vi "ToBoolean.vi"(8 "error in":errorcluster, 11 "Generic in":refnum<class "Generic.lvclass">) -> (0 "error out":errorcluster, 3 "Boolean out":refnum<class "Boolean.lvclass">)   [LabVIEW 2014, in "Boolean.lvclass"]
uses:
  Boolean.lvclass
  Generic/Generic.lvclass
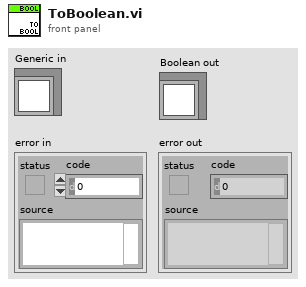
[diagram p1: front panel]
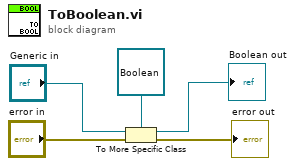
[diagram p0: block diagram]
diagram:
  n1 = To More Specific Class(target class=refnum<class "Boolean.lvclass"> refnum ("Boolean out"), reference="Generic in", error in="error in") -> (specific class reference=→"Boolean out":refnum<class "Boolean.lvclass">, error out=→"error out":errorcluster)
